vi "FluxRW_demo.vi"() -> ()   [LabVIEW 2019]
panel:
  in  "Write":bool
  in  "stop":bool
  out "Data Read Graph":dbl(graph)
  in  "Função de Leitura":i32(ring)=2 items=["Zero in progress", "Perform flowmeter zeroing", "Mass flow rate", "Density", "Temperature", "Volume flow rate", "Pressure (internally derived)", "Mass total", "Volume total", "Mass inventory", "Volume inventory", "Start/stop all totalizers", "Reset all totalizers", "Reset all inventories", "Real-time interrupt failure", "Sensor failure", "Temperature sensor failure", "Flowmeter zeroing failure", "Other failure occurred", "Mass flow rate meter factor", "Volume flow rate meter factor", "Density meter factor", "Flowing density calibration constant", "Mass flow scale factor", "Density scale factor", "Temperature scale factor", "Volume flow scale factor", "Pressure scale factor", "Mass total scale factor", "Volume total scale factor", "Mass inventory scale factor", "Volume inventory scale factor", "Flowmeter zeroing standard deviantion (units in microsec)", "Standard or special mass flow unit", "Density unit", "Temperature unit", "Standard or special volume flow unit", "Pressure unit", "Standard or special mass total or inventory unit", "Standard or special volume total or inventory unit", "Base mass unit for special mass unit", "Base time uni for special mass unit", "Base volume unit for special volume unit", "Base time unit for special volume unit", "Maximum zeroing time", "Flow direction", "EEProm checksum failure", "EEProm checksum failure in core processor", "EEProm database corrupt", "RAM diagnostic failure", "RAM diagnostic failure in core processor", "Real-time Interrupt failure", "Watchdog timer error", "Mass flow cutoff", "Volume flow cutoff", "Integer de erro 001", "Slug flow high-density limit (g/cm3)", "Slug flow low-density limit (g/cm3)"]
  in  "Data Write":dbl
  in  "Função de Escrita":i32(ring) items=["Perform flowmeter zeroing", "Start/stop all totalizers", "Reset all totalizers", "Reset all inventories", "Mass flow rate meter factor", "Volume flow rate meter factor", "Density meter factor", "Flowing density calibration constant", "Mass flow scale factor", "Density scale factor", "Temperature scale factor", "Volume flow scale factor", "Pressure scale factor", "Mass total scale factor", "Volume total scale factor", "Mass inventory scale factor", "Volume inventory scale factor", "Standard or special mass flow unit", "Density unit", "Temperature unit", "Standard or special volume flow unit", "Pressure unit", "Standard or special mass total or inventory unit", "Standard or special volume total or inventory unit", "Base mass unit for special mass unit", "Base time uni for special mass unit", "Base volume unit for special volume unit", "Base time unit for special volume unit", "Maximum zeroing time", "Flow direction", "Perform transmitter self-test", "Mass flow cutoff", "Volume flow cutoff", "Slug flow high-density limit (g/cm3)", "Slug flow low-density limit (g/cm3)"]
  out "Erro Fluximetro":errorcluster
  out "Data Read":dbl
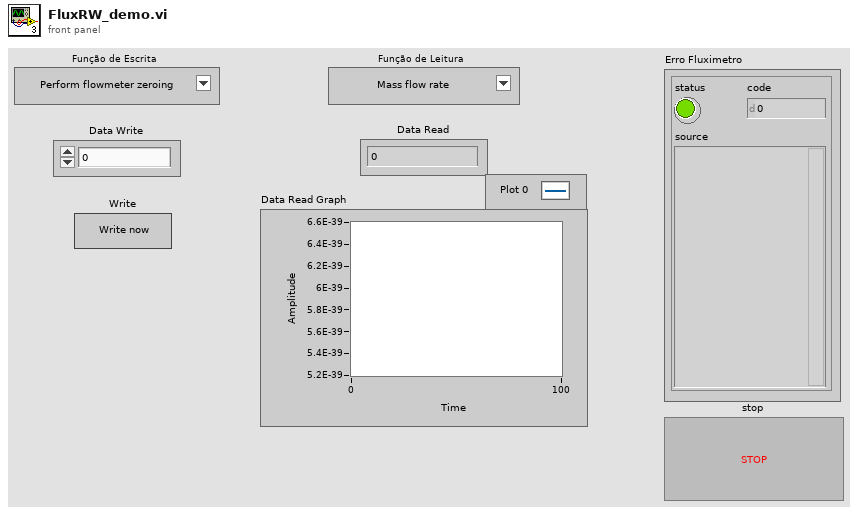
[diagram p1: front panel]
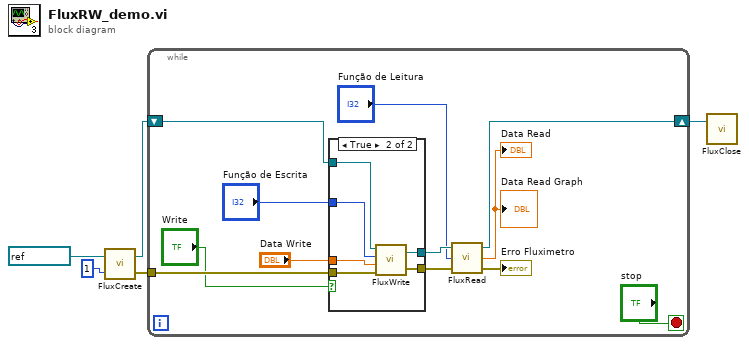
[diagram p0: block diagram]
diagram:
  n1 = call "FluxCreate.vi"("Endereço slave"=u16 1, "Recurso VISA"=refnum<visa-resource-name> "COM3" ("VISA resource")) -> ("Error Out"=w1:errorcluster, "Master Out"=w3:refnum<class "Modbus Master.lvclass">)
  n2 = while {
    shift-right: [w14] -> w2
    shift-left: w3 -> [w16]
    tunnel: w1 -> [w9]
    stop <- "stop" stop-if-true
    n3 = case shown="True" "Write" {
      tunnel: w16 -> [w19 w25]
      tunnel: [w19 w24] -> w15
      tunnel: "Função de Escrita" -> [_ w23]
      tunnel: "Data Write" -> [_ w22]
      tunnel: w9 -> [w18 w21]
      tunnel: [w18 w20] -> w8
      frame False {
      }
      frame True {
        n4 = call "FluxWrite.vi"("Error In"=w21, "Data"=w22, "Função de Escrita"=w23, "Master In"=w25) -> ("Error Out"=w20:errorcluster, "Master Out"=w24:refnum<class "Modbus Master.lvclass">)
      }
    }
    n5 = call "FluxRead.vi"("Error In"=w8, "Função de Leitura"="Função de Leitura", "Master In"=w15) -> ("Error Out"=→"Erro Fluximetro":errorcluster, "Data"=→"Data Read" →"Data Read Graph":dbl, "Master Out"=w14:refnum<class "Modbus Master.lvclass">)
  }
  n6 = call "FluxClose.vi"("Master In"=w2) -> ()  [unwired: 1 in, 1 out]
